vi "Configure.vi"(8 "error in":errorcluster, 10 "name":string, 11 "Instrument in":refnum<class "Instrument.lvclass">) -> (0 "error out":errorcluster, 3 "Instrument out":refnum<class "Instrument.lvclass">)   [LabVIEW 2015, in "Instrument.lvclass"]
doc: "Configure the Instrument object. The default behavior is to provide a name and define a command enqueuer."
uses:
  Instrument.lvclass
  Commands/Command.lvclass
  Instrument.lvclass/Instrument.ctl
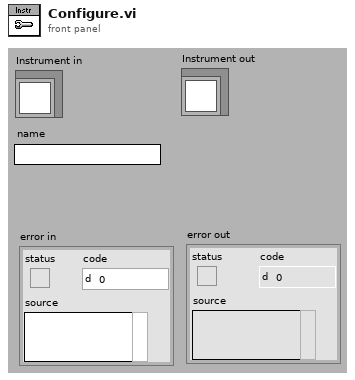
[diagram p1: front panel]
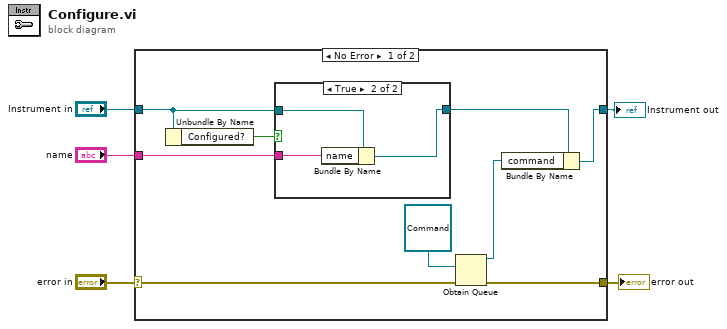
[diagram p0: block diagram]
diagram:
  n1 = case shown="No Error" "error in" {
    selector: "error in" -> [w8 w20]
    tunnel: [w7 w20] -> w4
    tunnel: [w6 w19] -> w2
    tunnel: "Instrument in" -> [w13 w19]
    tunnel: "name" -> [w14 _]
    frame No Error {
      n2 = Unbundle By Name(w13) -> ("Configured?"=w12:bool)
      n3 = case shown="True" w12 {
        tunnel: [w15 w18] -> w11
        tunnel: w13 -> [w15 w17]
        tunnel: w14 -> [_ w16]
        frame False {
        }
        frame True {
          n4 = Bundle By Name(cluster=w17, "name"=w16) -> (w18:refnum<class "Instrument.lvclass">)
        }
      }
      n5 = Obtain Queue(element data type=refnum<class "Command.lvclass"> refnum ("Command"), error in (no error)=w8) -> (queue out=w9:refnum<queue>, error out=w7:errorcluster)  [unwired: 3 in, 1 out]
      n6 = Bundle By Name(cluster=w11, "command"=w9) -> (w6:refnum<class "Instrument.lvclass">)
    }
    frame Error {
    }
  }
  "error out" <- w4
  "Instrument out" <- w2
